vi "DC_CNTRL_fast_select_module_and_change_potential.vi"(0 "Handle":u64, 1 "Current Potential (V)":dbl, 2 "Target Potential (V)":dbl, 3 "Max Potential (V)":dbl, 5 "Box Number":u16(ring), 7 "Current Module Number":u16(ring) items=["0", "1", "2", "3", "4", "5", "6", "7"], 9 "Desired Module Number":u16(ring) items=["0", "1", "2", "3", "4", "5", "6", "7"], 11 "error in (no error)":errorcluster) -> (4 "Handle out":u64, 13 "Current Module Number Out":u16, 15 "error out":errorcluster)   [LabVIEW 2019]
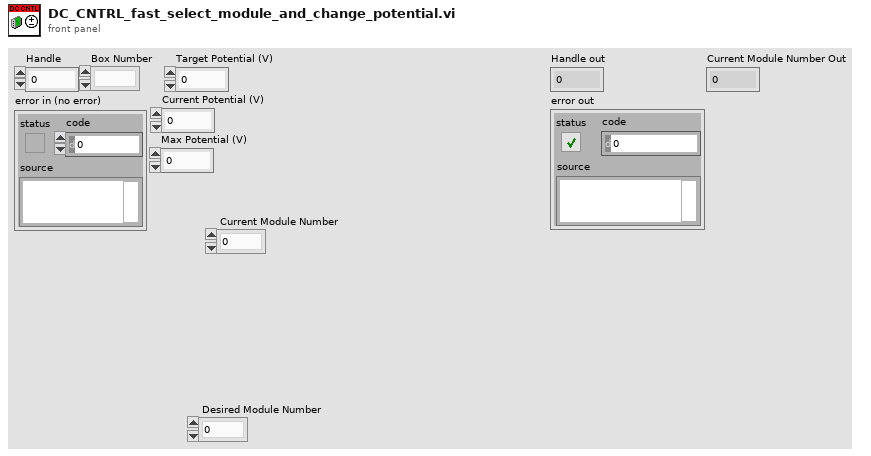
[diagram p1: front panel]
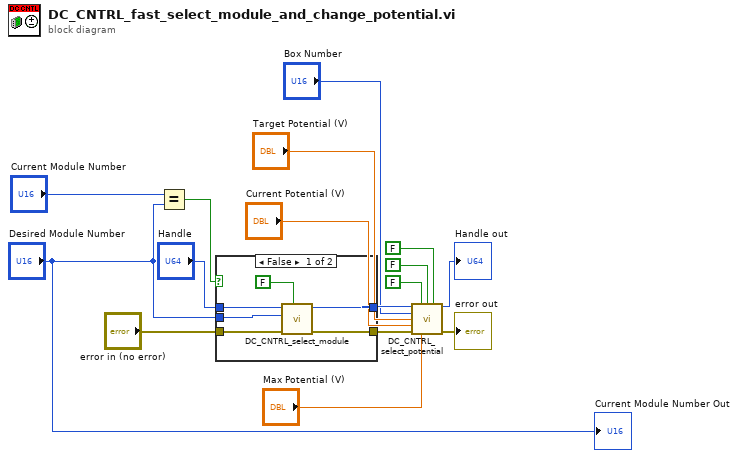
[diagram p0: block diagram]
diagram:
  n1 = Equal?(x="Current Module Number", y="Desired Module Number") -> (x = y?=w3:bool)
  n2 = case shown="False" w3 {
    tunnel: "Handle" -> [w22 w24]
    tunnel: "error in (no error)" -> [w21 w23]
    tunnel: [w19 w24] -> w14
    tunnel: [w18 w23] -> w13
    tunnel: "Desired Module Number" -> [w17 _]
    frame False {
      n3 = call "DC_CNTRL_select_module.vi"("Read Answer?"=FALSE, "error in (no error)"=w21, "Module number"=w17, "Handle"=w22) -> ("error out"=w18:errorcluster, "Handle out"=w19:u64)  [unwired: 6 in]
    }
    frame True {
    }
  }
  n4 = call "DC_CNTRL_select_potential.vi"("Handle"=w14, "Ignore NACK"=FALSE, "Read Answer?"=FALSE, "Clear  RxTx Buffer?"=FALSE, "Box Number"="Box Number", "Target Potential (V)"="Target Potential (V)", "Current Potential (V)"="Current Potential (V)", "error in (no error)"=w13, "Max Potential (V)"="Max Potential (V)") -> ("Handle out"=→"Handle out":u64, "error out"=→"error out":errorcluster)  [unwired: 5 in]
  "Current Module Number Out" <- "Desired Module Number"
